vi "BooleanBehaviors.vi"() -> ()   [LabVIEW 2014]
uses:
  <vilib>/event_ctls.llb/lveventtype.ctl
panel:
  out "Mechanical Action:":u32(ring) items=["Switch When Pressed", "Switch When Released", "Switch Until Released", "Latch When Pressed", "Latch When Released", "Latch Until Released"]
  out "History":i16(graph)
  out "L Mouse Down":bool
  in  "stop":bool
  out "Reading Terminal":bool
  out "State":bool
  in  "Boolean":bool
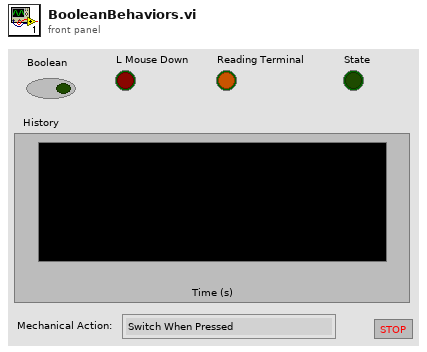
[diagram p1: front panel]
types:
  T1 = typedef "lveventtype.ctl" = enum32{"Null", "Timeout", "Annotation Menu Selection", "Annotation Menu Selection?", "App Instance Close", "App Instance Close?", "Autoscale Range Change", "Bookmark Info Change", "Cell Edit", "Cell Edit?", "Cursor Grab", "Cursor Grab?", "Cursor Menu Selection", "Cursor Menu Selection?", "Cursor Move", "Cursor Release", "Data Change", "Direction Change", "Display State Change", "Drag Ended", "Drag Enter", "Drag Leave", "Drag Over", "Drag Source Update", "Drag Starting", "Drag Starting?", "Drop", "Exec State Change", "Key Down", "Key Down?", "Key Repeat", "Key Repeat?", "Key Up", "Listbox Double Click", "Menu Activation?", "Menu Selection (App)", "Menu Selection? (App)", "Menu Selection (User)", "Mouse Down", "Mouse Down?", "Mouse Enter", "Mouse Leave", "Mouse Move", "Mouse Up", "Mouse Wheel", "NI Security User Change (App)", "Pane Size", "Panel Close", "Panel Close?", "Panel Resize", "Plot Attribute Change", "Scale Range Change", "Shortcut Menu Activation?", "Shortcut Menu Selection (App)", "Shortcut Menu Selection? (App)", "Shortcut Menu Selection (User)", "Tree Double Click", "Tree Drag", "Tree Drag?", "Tree Drop", "Tree Drop?", "Tree Item Close", "Tree Item Close?", "Tree Item Open", "Tree Item Open?", "User Event", "Value Change"}
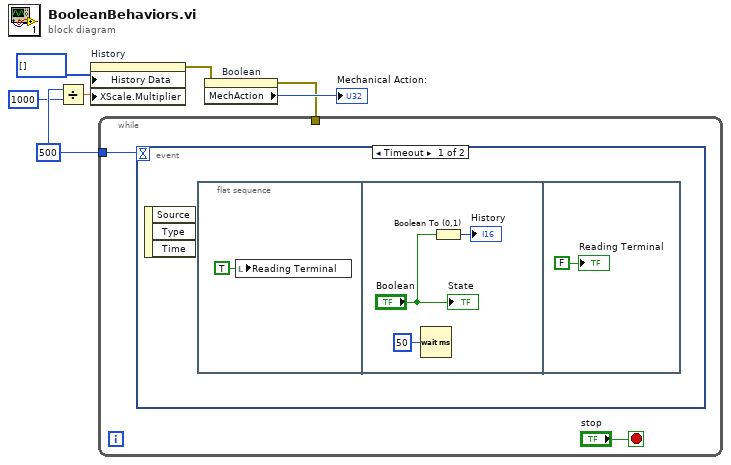
[diagram p0: block diagram]
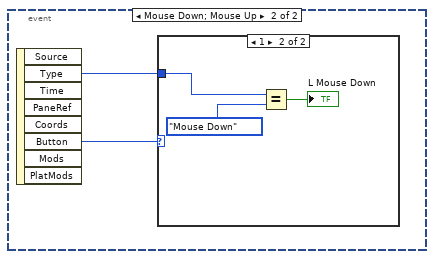
[diagram p2: hidden frame]
diagram:
  w7 = 500
  n1 = Divide(x=w7, y=1000) -> (x/y=w5:dbl)
  n2 = property on="History" class="WFChart (strict)"("History Data"=i16[] [], "XScale.Multiplier"=w5) -> (error out=w4:errorcluster)  [unwired: 2 in, 1 out]
  n3 = property on="Boolean" class="Bool (strict)"(error in=w4) -> (error out=w2:errorcluster, "MechAction"=→"Mechanical Action:":u32)  [unwired: 1 in, 1 out]
  n4 = while {
    tunnel: w7 -> [w8]
    tunnel: w2 -> [_]
    stop <- "stop" stop-if-true
    n5 = event shown="[0] Timeout" {
      selector: _ -> [_ _]
      dyn-events: _ -> [_ _]
      timeout: w8 -> [_ _]
      event Timeout {
        n6 = event-data() -> ()  [unwired: 1 in, 3 out]
        n7 = flat-sequence {
          frame #0 {
            n8 = local write "Reading Terminal"(TRUE ("Reading Terminal")) -> ()
          }
          frame #1 {
            n9 = Wait (ms)(milliseconds to wait=u32 50) -> ()  [unwired: 1 out]
            n10 = Boolean To (0,1)(Boolean="Boolean") -> (0, 1=→"History":i16)
            "State" <- "Boolean"
          }
          frame #2 {
            "Reading Terminal" <- FALSE ("Reading Terminal")
          }
        }
      }
      event Mouse Down; Mouse Up {
        n11 = event-data() -> ("Type"=w15:T1, "Button"=w16:u16)  [unwired: 1 in, 6 out]
        n12 = case shown="1" w16 {
          tunnel: w15 -> [_ w19]
          frame 0, Default {
          }
          frame 1 {
            n13 = Equal?(x=w19, y=lveventtype."Mouse Down") -> (x = y?=→"L Mouse Down":bool)
          }
        }
      }
    }
  }
